vi "Begin.vi"(8 "error in":errorcluster) -> (0 "error out":errorcluster)   [LabVIEW 2018]
doc: "Called before other user functions, this VI is expected to open initial I/O refnums, load in file data, and do all program initialization. Notice that the <B>error out</B> terminal is simply used for data flow. Wiring it to other structures or subVIs ensures that this VI runs first."
uses:
  <vilib>/Rock Robotics/WPI/DriverStation/WPI_DriverStationRobotMode2.ctl
  <vilib>/Rock Robotics/WPI/Joystick/WPI_JoystickDeviceEnum.ctl
  <vilib>/Rock Robotics/SystemInterfaces/DIO/FPGA_DIOChannel.ctl
  <vilib>/Rock Robotics/WPI/Solenoid/WPI_SolenoidChannel.ctl
  <vilib>/Rock Robotics/WPI/ThirdParty/Sensors/navX/_TypeDefs/FRIC_navX_DeviceNumbersTypeDef.ctl
  <vilib>/Rock Robotics/SystemInterfaces/AI/FPGA_AIChannel.ctl
  Robot Global Data.vi
  <vilib>/Rock Robotics/WPI/Counter/WPI_CounterDigitalInputToDigitalSource.vi
  <vilib>/Rock Robotics/WPI/Solenoid/WPI_SolenoidOpenSingle.vi
  <vilib>/Rock Robotics/WPI/Utilities/WPI_GetSetVariantRefNum.vi
  <vilib>/Rock Robotics/WPI/Switch/WPI_SwitchOpenLimit.vi
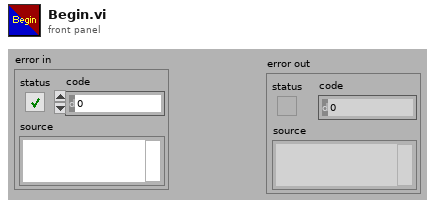
[diagram p1: front panel]
types:
  T1 = typedef "WPI_SolenoidChannel.ctl" = enum8{"Solenoid 0", "Solenoid 1", "Solenoid 2", "Solenoid 3", "Solenoid 4", "Solenoid 5", "Solenoid 6", "Solenoid 7", "Invalid"}
  T2 = typedef "FPGA_AIChannel.ctl" = enum8{"AI 0", "AI 1", "AI 2", "AI 3", "AI MXP 0", "AI MXP 1", "AI MXP 2", "AI MXP 3", "Invalid"}
  T3 = typedef "FRIC_navX_DeviceNumbersTypeDef.ctl" = enum16{"Dev0", "Dev1", "Dev2", "Dev3"}
  T4 = typedef "FPGA_DIOChannel.ctl" = enum8{"DIO 0", "DIO 1", "DIO 2", "DIO 3", "DIO 4", "DIO 5", "DIO 6", "DIO 7", "DIO 8", "DIO 9", "DIO MXP 0", "DIO MXP 1", "DIO MXP 2", "DIO MXP 3", "DIO MXP 4", "DIO MXP 5", "DIO MXP 6", "DIO MXP 7", "DIO MXP 8", "DIO MXP 9", "DIO MXP 10", "DIO MXP 11", "DIO MXP 12", "DIO MXP 13", "DIO MXP 14", "DIO MXP 15", "SPI Port CS1", "SPI Port CS2", "SPI Port CS3", "SPI Port MISO", "SPI Port MOSI", "Invalid"}
  T5 = typedef "WPI_JoystickDeviceEnum.ctl" = enum16{"USB 0", "USB 1", "USB 2", "USB 3", "USB 4", "USB 5"}
  T6 = typedef "WPI_DriverStationRobotMode2.ctl" = enum16{"Autonomous Disabled", "Autonomous Enabled", "Teleop Disabled", "Teleop Enabled", "Disconnected", "Finish", "Test Disabled", "Test Enabled", "Emergency Stopped"}
  T7 = typedef "WPI_DigitalInputDevRef.ctl" = cluster{"DevStatus":errorcluster, "DIO Channel":T4}
  T8 = typedef "FPGA_CounterEncoderSourceConvertionLVSourceType.ctl" = cluster{"DevStatus":errorcluster, "AnalogTriggerMode?":bool, "DigitalMode":cluster{"DIO Channel":T9}, "AnalogTriggerMode":cluster{"AnalogTriggerIndex":T10, "OutputType":T11}}
  T9 = typedef "FPGA_DIODigitalSourceChannel.ctl" = enum8{"DIO 0", "DIO 1", "DIO 2", "DIO 3", "DIO 4", "DIO 5", "DIO 6", "DIO 7", "DIO 8", "DIO 9", "DIO MXP 0", "DIO MXP 1", "DIO MXP 2", "DIO MXP 3", "DIO MXP 4", "DIO MXP 5", "DIO MXP 6", "DIO MXP 7", "DIO MXP 8", "DIO MXP 9", "DIO MXP 10", "DIO MXP 11", "DIO MXP 12", "DIO MXP 13", "DIO MXP 14", "DIO MXP 15", "SPI Port CS1", "SPI Port CS2", "SPI Port CS3", "SPI Port MISO", "SPI Port MOSI", "Disabled"}
  T10 = typedef "FPGA_AnalogTriggerIndex.ctl" = enum8{"Trig 0", "Trig 1", "Trig 2", "Trig 3", "Trig 4", "Trig 5", "Trig 6", "Trig 7", "Invalid"}
  T11 = typedef "FPGA_AnalogTriggerOutType.ctl" = enum16{"InWindow", "TriggerState", "Rising", "Falling"}
  T12 = typedef "WPI_EncoderDevRef.ctl" = cluster{"DevStatus":errorcluster, "EncoderIndex":T13, "CounterIndex":T14, "DistancePerCount":dbl, "Decoding Type":T15}
  T13 = typedef "FPGA_EncoderIdx.ctl" = enum8{"Enc 0", "Enc 1", "Enc 2", "Enc 3", "Enc 4", "Enc 5", "Enc 6", "Enc 7", "Invalid"}
  T14 = typedef "FPGA_CounterCtrSystemIndex.ctl" = enum8{"Ctr 0", "Ctr 1", "Ctr 2", "Ctr 3", "Ctr 4", "Ctr 5", "Ctr 6", "Ctr 7", "Invalid"}
  T15 = typedef "WPI_EncoderType.ctl" = enum16{"1x", "2x", "4x"}
  T16 = typedef "WPI_JoystickDevRef.ctl" = cluster{"Device":T5}
  T17 = typedef "WPI_MotorControlDeviceRef.ctl" = cluster{"DeviceStatus":errorcluster, "Type":T18, "PWM":cluster{"PWM Channel":T19, "DeadBand":T20}, "CAN":cluster{"Device Number":u8, "SetOutput VI Ref":variant, "GetOutput VI Ref":variant, "Enable VI Ref":variant, "Disable VI Ref":variant, "Data":variant}, "Invert":bool, "DIO PWM":cluster{"PWM \"Enable\" Channel":T19, "DIOChannel":T4, "PWM Rate":dbl}}
  T18 = typedef "WPI_MotorControlType.ctl" = enum16{"PWM", "CAN", "DIO PWM"}
  T19 = typedef "FPGA_DIOPWMChannel.ctl" = enum8{"PWM 0", "PWM 1", "PWM 2", "PWM 3", "PWM 4", "PWM 5", "PWM 6", "PWM 7", "PWM 8", "PWM 9", "PWM MXP 0", "PWM MXP 1", "PWM MXP 2", "PWM MXP 3", "PWM MXP 4", "PWM MXP 5", "PWM MXP 6", "PWM MXP 7", "PWM MXP 8", "PWM MXP 9", "Invalid"}
  T20 = typedef "WPI_PWMDeadband.ctl" = cluster{"Name":string, "maxPositivePwm":i32, "minPositivePwm":i32, "centerPwm":i32, "maxNegativePwm":i32, "minNegativePwm":i32, "angularRange":u16}
  T21 = typedef "WPI_CompressorDevRef.ctl" = cluster{"DevStatus":errorcluster, "Pneumatics Control Module":u8}
  T22 = typedef "WPI_SolenoidDevRef.ctl" = cluster{"DevStatus":errorcluster, "Pneumatics Control Module":u8, "Forward Solenoid Channel":T1, "Reverse Solenoid Channel":T1}
  T23 = typedef "WPI_SwitchDevRef.ctl" = cluster{"DevStatus":errorcluster, "DIO Channel":T4, "CntIndex":T14, "Normally Closed":bool}
  T24 = typedef "WPI_PotentiometerDevRef.ctl" = cluster{"DevStatus":errorcluster, "Analog Channel":T2, "Invert Output":bool}
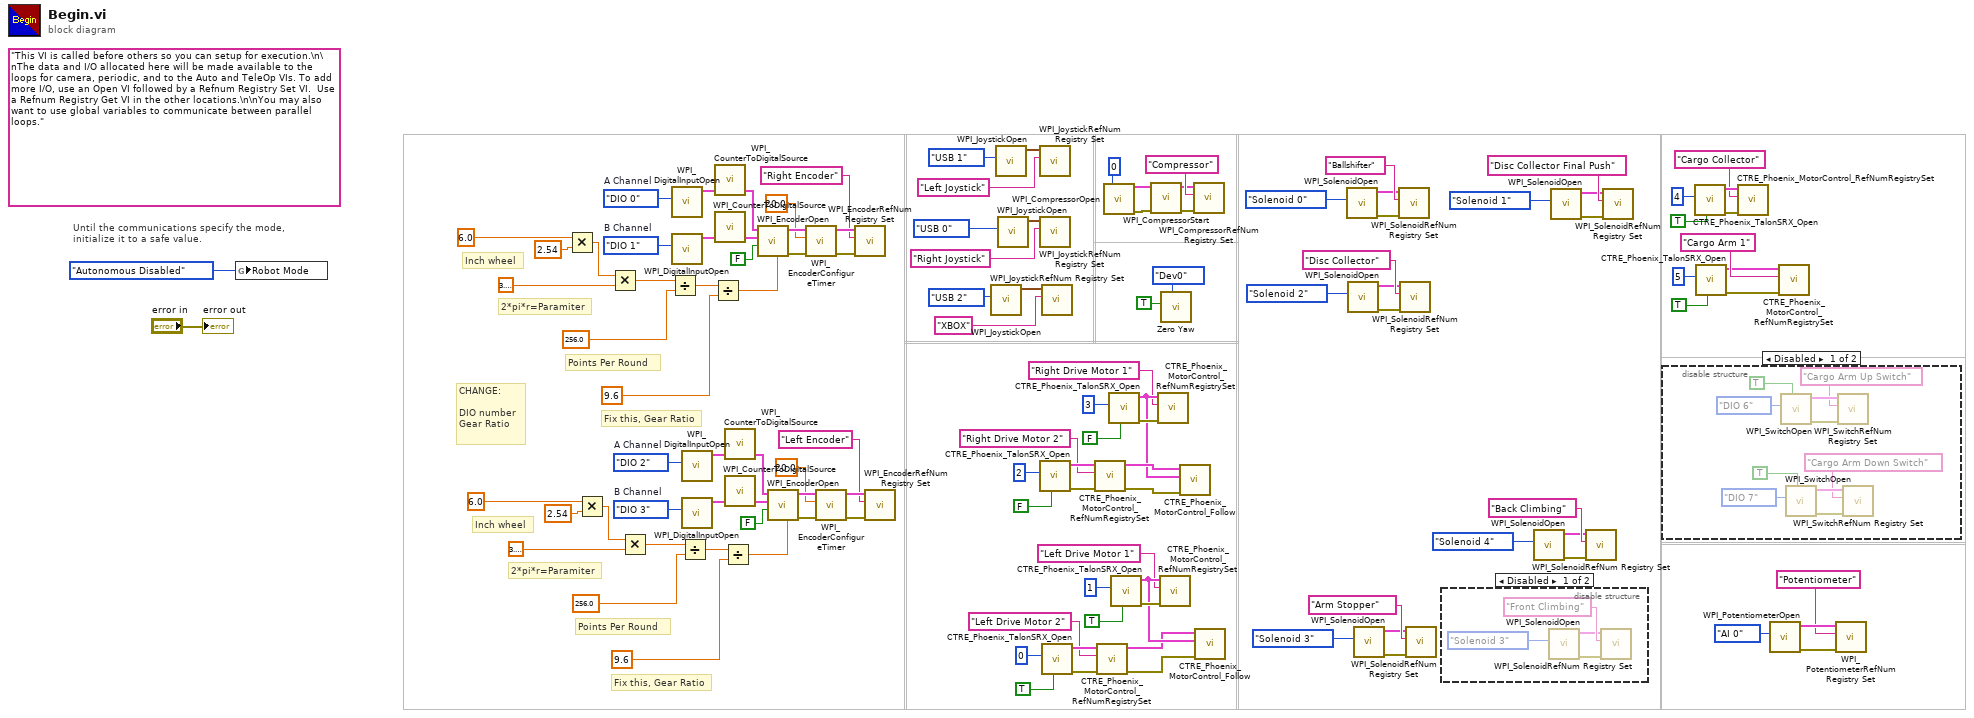
[diagram p0: block diagram]
diagram:
  w89 = FPGA_DIOChannel."DIO 3"  # B Channel
  w88 = FPGA_DIOChannel."DIO 2"  # A Channel
  w111 = FPGA_DIOChannel."DIO 1"  # B Channel
  w110 = FPGA_DIOChannel."DIO 0"  # A Channel
  (unwired) "This VI is called before others so you can setup for execution.\n\nThe data and I/O allocated here will be made available to the loops for camera, periodic, and to the Auto and TeleOp VIs. To add more I/O, use an Open VI followed by a Refnum Registry Set VI.  Use a Refnum Registry Get VI in the other locations.\n\nYou may also want to use global variables to communicate between parallel loops."
  # "CHANGE: \n\nDIO number\nGear Ratio"
  # "2*pi*r=Paramiter"
  # "Points Per Round"
  # "Inch wheel"
  # "Fix this, Gear Ratio"
  # "2*pi*r=Paramiter"
  # "Points Per Round"
  # "Inch wheel"
  # "Fix this, Gear Ratio"
  # "Until the communications specify the mode,\ninitialize it to a safe value."
  n1 = global write "Robot Global Data.vi" "Robot Mode"(WPI_DriverStationRobotMode2."Autonomous Disabled" ("Robot Mode")) -> ()
  n2 = Multiply(x=6.0, y=2.54) -> (x*y=w98:dbl)
  n3 = Multiply(x=6.0, y=2.54) -> (x*y=w76:dbl)
  n4 = Multiply(x=w98, y=3.141592653589793) -> (x*y=w96:dbl)
  n5 = Multiply(x=w76, y=3.141592653589793) -> (x*y=w74:dbl)
  n6 = Divide(x=w96, y=256.0) -> (x/y=w94:dbl)
  n7 = call <vilib>:"WPI_DigitalInputOpen.vi"("DIO Channel"=w110) -> ("DigitalInputDevRef"=w107:T7)  [unwired: 1 in, 9 out]
  n8 = call <vilib>:"WPI_DigitalInputOpen.vi"("DIO Channel"=w111) -> ("DigitalInputDevRef"=w108:T7)  [unwired: 1 in, 9 out]
  n9 = Divide(x=w74, y=256.0) -> (x/y=w72:dbl)
  n10 = call <vilib>:"WPI_DigitalInputOpen.vi"("DIO Channel"=w88) -> ("DigitalInputDevRef"=w85:T7)  [unwired: 1 in, 9 out]
  n11 = call <vilib>:"WPI_DigitalInputOpen.vi"("DIO Channel"=w89) -> ("DigitalInputDevRef"=w86:T7)  [unwired: 1 in, 9 out]
  n12 = Divide(x=w94, y=9.6) -> (x/y=w92:dbl)
  n13 = call-poly <vilib>:"WPI_CounterToDigitalSource.vi"("DigitalInputDevRef"=w107) -> ("Digital Source"=w106:T8)  [unwired: 6 out]
  n14 = call-poly <vilib>:"WPI_CounterToDigitalSource.vi"("DigitalInputDevRef"=w108) -> ("Digital Source"=w109:T8)  [unwired: 6 out]
  n15 = Divide(x=w72, y=9.6) -> (x/y=w70:dbl)
  n16 = call-poly <vilib>:"WPI_CounterToDigitalSource.vi"("DigitalInputDevRef"=w85) -> ("Digital Source"=w84:T8)  [unwired: 6 out]
  n17 = call-poly <vilib>:"WPI_CounterToDigitalSource.vi"("DigitalInputDevRef"=w86) -> ("Digital Source"=w87:T8)  [unwired: 6 out]
  n18 = call <vilib>:"WPI_EncoderOpen.vi"("DistancePerCount"=w92, "Invert Direction (False)"=FALSE, "BSource"=w109, "ASource"=w106) -> ("error out"=w105:errorcluster, "EncoderDevRef"=w104:T12)  [unwired: 4 in, 2 out]
  n19 = call <vilib>:"WPI_EncoderOpen.vi"("DistancePerCount"=w70, "Invert Direction (False)"=FALSE, "BSource"=w87, "ASource"=w84) -> ("error out"=w83:errorcluster, "EncoderDevRef"=w82:T12)  [unwired: 4 in, 2 out]
  n20 = call <vilib>:"WPI_EncoderConfigureTimer.vi"("error in (no error)"=w105, "Minimum Rate"=20.0, "EncoderDevRef"=w104) -> ("error out"=w102:errorcluster, "EncoderDevRef"=w103:T12)  [unwired: 7 in]
  n21 = call <vilib>:"WPI_EncoderConfigureTimer.vi"("error in (no error)"=w83, "Minimum Rate"=20.0, "EncoderDevRef"=w82) -> ("error out"=w80:errorcluster, "EncoderDevRef"=w81:T12)  [unwired: 7 in]
  n22 = call <vilib>:"WPI_EncoderRefNum Registry Set.vi"("error in (no error)"=w102, "refnum name"="Right Encoder", "EncoderDevRef"=w103) -> ()  [unwired: 7 in, 2 out]
  n23 = call <vilib>:"WPI_EncoderRefNum Registry Set.vi"("error in (no error)"=w80, "refnum name"="Left Encoder", "EncoderDevRef"=w81) -> ()  [unwired: 7 in, 2 out]
  n24 = call <vilib>:"WPI_JoystickOpen.vi"("JoystickDevice"=WPI_JoystickDeviceEnum."USB 2") -> ("JoystickDevRef"=w120:T16)  [unwired: 10 in]
  n25 = call <vilib>:"WPI_JoystickOpen.vi"("JoystickDevice"=WPI_JoystickDeviceEnum."USB 1") -> ("JoystickDevRef"=w113:T16)  [unwired: 10 in]
  n26 = call <vilib>:"WPI_JoystickOpen.vi"("JoystickDevice"=WPI_JoystickDeviceEnum."USB 0") -> ("JoystickDevRef"=w116:T16)  [unwired: 10 in]
  n27 = call <vilib>:"WPI_JoystickRefNum Registry Set.vi"("refnum name"="Left Joystick", "JoystickDevRef"=w113) -> ()  [unwired: 8 in, 2 out]
  n28 = call <vilib>:"WPI_JoystickRefNum Registry Set.vi"("refnum name"="Right Joystick", "JoystickDevRef"=w116) -> ()  [unwired: 8 in, 2 out]
  n29 = call <vilib>:"CTRE_Phoenix_TalonSRX_Open.vi"("Invert"=FALSE, "Device Number"=u8 2) -> ("error out"=w44:errorcluster, "CAN Talon SRX Ref"=w53:T17)  [unwired: 8 in]
  n30 = call <vilib>:"WPI_JoystickRefNum Registry Set.vi"("refnum name"="XBOX", "JoystickDevRef"=w120) -> ()  [unwired: 8 in, 2 out]
  n31 = call <vilib>:"CTRE_Phoenix_TalonSRX_Open.vi"("Invert"=TRUE, "Device Number"=u8 0) -> ("error out"=w64:errorcluster, "CAN Talon SRX Ref"=w65:T17)  [unwired: 8 in]
  n32 = call <vilib>:"CTRE_Phoenix_MotorControl_RefNumRegistrySet.vi"("error in (no error)"=w44, "refnum name"="Right Drive Motor 2", "PhoenixMotorControlDevRef"=w53) -> ("error out"=w45:errorcluster, "PhoenixMotorControlDevRef"=w52:T17)  [unwired: 7 in]
  n33 = call <vilib>:"CTRE_Phoenix_MotorControl_RefNumRegistrySet.vi"("error in (no error)"=w64, "refnum name"="Left Drive Motor 2", "PhoenixMotorControlDevRef"=w65) -> ("error out"=w46:errorcluster, "PhoenixMotorControlDevRef"=w59:T17)  [unwired: 7 in]
  n34 = call <vilib>:"WPI_CompressorOpen.vi"("Pneumatics Control Module (0)"=u8 0) -> ("CompressorDevRef"=w8:T21, "error out"=w6:errorcluster)  [unwired: 13 in]
  n35 = call <vilib>:"CTRE_Phoenix_TalonSRX_Open.vi"("Invert"=FALSE, "Device Number"=u8 3) -> ("error out"=w54:errorcluster, "CAN Talon SRX Ref"=w51:T17)  [unwired: 8 in]
  n36 = call <vilib>:"CTRE_Phoenix_TalonSRX_Open.vi"("Invert"=TRUE, "Device Number"=u8 1) -> ("error out"=w67:errorcluster, "CAN Talon SRX Ref"=w60:T17)  [unwired: 8 in]
  n37 = call <vilib>:"WPI_CompressorStart.vi"("error in (no error)"=w6, "CompressorDevRef"=w8) -> ("error out"=w5:errorcluster, "CompressorDevRef"=w7:T21)  [unwired: 8 in]
  n38 = call <vilib>:"CTRE_Phoenix_MotorControl_RefNumRegistrySet.vi"("error in (no error)"=w54, "refnum name"="Right Drive Motor 1", "PhoenixMotorControlDevRef"=w51) -> ()  [unwired: 7 in, 2 out]
  n39 = call <vilib>:"CTRE_Phoenix_MotorControl_RefNumRegistrySet.vi"("error in (no error)"=w67, "refnum name"="Left Drive Motor 1", "PhoenixMotorControlDevRef"=w60) -> ()  [unwired: 7 in, 2 out]
  n40 = call <vilib>:"Zero Yaw.vi"("Device Number"=FRIC_navX_DeviceNumbersTypeDef."Dev0", "Zero"=TRUE) -> ()  [unwired: 10 in]
  n41 = call <vilib>:"CTRE_Phoenix_MotorControl_Follow.vi"("error in (no error)"=w45, "Master Controller to Follow"=w51, "PhoenixMotorControlDevRef"=w52) -> ()  [unwired: 7 in, 2 out]
  n42 = call <vilib>:"WPI_CompressorRefNum Registry Set.vi"("error in (no error)"=w5, "refnum name"="Compressor", "CompressorDevRef"=w7) -> ()  [unwired: 7 in, 2 out]
  n43 = call <vilib>:"CTRE_Phoenix_MotorControl_Follow.vi"("error in (no error)"=w46, "Master Controller to Follow"=w60, "PhoenixMotorControlDevRef"=w59) -> ()  [unwired: 7 in, 2 out]
  n44 = call-poly <vilib>:"WPI_SolenoidOpen.vi"("Solenoid Channel"=WPI_SolenoidChannel."Solenoid 0") -> ("error out"=w39:errorcluster, "SolenoidDevRef"=w40:T22)  [unwired: 9 in]
  n45 = call-poly <vilib>:"WPI_SolenoidOpen.vi"("Solenoid Channel"=WPI_SolenoidChannel."Solenoid 2") -> ("error out"=w35:errorcluster, "SolenoidDevRef"=w36:T22)  [unwired: 9 in]
  n46 = call-poly <vilib>:"WPI_SolenoidOpen.vi"("Solenoid Channel"=WPI_SolenoidChannel."Solenoid 3") -> ("error out"=w1:errorcluster, "SolenoidDevRef"=w2:T22)  [unwired: 9 in]
  n47 = call <vilib>:"WPI_SolenoidRefNum Registry Set.vi"("error in (no error)"=w39, "refnum name"="Ballshifter", "SolenoidDevRef"=w40) -> ()  [unwired: 7 in, 2 out]
  n48 = call <vilib>:"WPI_SolenoidRefNum Registry Set.vi"("error in (no error)"=w35, "refnum name"="Disc Collector", "SolenoidDevRef"=w36) -> ()  [unwired: 7 in, 2 out]
  n49 = call <vilib>:"WPI_SolenoidRefNum Registry Set.vi"("error in (no error)"=w1, "refnum name"="Arm Stopper", "SolenoidDevRef"=w2) -> ()  [unwired: 7 in, 2 out]
  n50 = disable-structure shown="Disabled" {
    frame Disabled {
      n51 = call-poly <vilib>:"WPI_SolenoidOpen.vi"("Solenoid Channel"=WPI_SolenoidChannel."Solenoid 3") -> ("error out"=w122:errorcluster, "SolenoidDevRef"=w123:T22)  [unwired: 9 in]
      n52 = call <vilib>:"WPI_SolenoidRefNum Registry Set.vi"("error in (no error)"=w122, "refnum name"="Front Climbing", "SolenoidDevRef"=w123) -> ()  [unwired: 7 in, 2 out]
    }
    frame Enabled {
    }
  }
  n53 = call-poly <vilib>:"WPI_SolenoidOpen.vi"("Solenoid Channel"=WPI_SolenoidChannel."Solenoid 4") -> ("error out"=w11:errorcluster, "SolenoidDevRef"=w12:T22)  [unwired: 9 in]
  n54 = call-poly <vilib>:"WPI_SolenoidOpen.vi"("Solenoid Channel"=WPI_SolenoidChannel."Solenoid 1") -> ("error out"=w24:errorcluster, "SolenoidDevRef"=w25:T22)  [unwired: 9 in]
  n55 = call <vilib>:"WPI_SolenoidRefNum Registry Set.vi"("error in (no error)"=w11, "refnum name"="Back Climbing", "SolenoidDevRef"=w12) -> ()  [unwired: 7 in, 2 out]
  n56 = call <vilib>:"WPI_SolenoidRefNum Registry Set.vi"("error in (no error)"=w24, "refnum name"="Disc Collector Final Push", "SolenoidDevRef"=w25) -> ()  [unwired: 7 in, 2 out]
  n57 = disable-structure shown="Disabled" {
    frame Disabled {
      n58 = call-poly <vilib>:"WPI_SwitchOpen.vi"("Normally Closed"=TRUE, "DIO Channel"=FPGA_DIOChannel."DIO 6") -> ("error out"=w135:errorcluster, "SwitchDevRef"=w134:T23)  [unwired: 8 in]
      n59 = call-poly <vilib>:"WPI_SwitchOpen.vi"("Normally Closed"=TRUE, "DIO Channel"=FPGA_DIOChannel."DIO 7") -> ("error out"=w132:errorcluster, "SwitchDevRef"=w131:T23)  [unwired: 8 in]
      n60 = call <vilib>:"WPI_SwitchRefNum Registry Set.vi"("error in (no error)"=w135, "refnum name"="Cargo Arm Up Switch", "SwitchDevRef"=w134) -> ()  [unwired: 7 in, 2 out]
      n61 = call <vilib>:"WPI_SwitchRefNum Registry Set.vi"("error in (no error)"=w132, "refnum name"="Cargo Arm Down Switch", "SwitchDevRef"=w131) -> ()  [unwired: 7 in, 2 out]
    }
    frame Enabled {
    }
  }
  n62 = call <vilib>:"CTRE_Phoenix_TalonSRX_Open.vi"("Invert"=TRUE, "Device Number"=u8 4) -> ("error out"=w33:errorcluster, "CAN Talon SRX Ref"=w34:T17)  [unwired: 8 in]
  n63 = call <vilib>:"CTRE_Phoenix_TalonSRX_Open.vi"("Invert"=TRUE, "Device Number"=u8 5) -> ("error out"=w30:errorcluster, "CAN Talon SRX Ref"=w23:T17)  [unwired: 8 in]
  n64 = call <vilib>:"CTRE_Phoenix_MotorControl_RefNumRegistrySet.vi"("error in (no error)"=w33, "refnum name"="Cargo Collector", "PhoenixMotorControlDevRef"=w34) -> ()  [unwired: 7 in, 2 out]
  n65 = call <vilib>:"WPI_PotentiometerOpen.vi"("Analog Channel"=FPGA_AIChannel."AI 0") -> ("error out"=w18:errorcluster, "PotDevRef"=w17:T24)  [unwired: 9 in]
  n66 = call <vilib>:"CTRE_Phoenix_MotorControl_RefNumRegistrySet.vi"("error in (no error)"=w30, "refnum name"="Cargo Arm 1", "PhoenixMotorControlDevRef"=w23) -> ()  [unwired: 7 in, 2 out]
  n67 = call <vilib>:"WPI_PotentiometerRefNum Registry Set.vi"("error in (no error)"=w18, "refnum name"="Potentiometer", "PotDevRef"=w17) -> ()  [unwired: 7 in, 2 out]
  "error out" <- "error in"
